vi "Save.vi"(8 "error in":errorcluster) -> (0 "error out":errorcluster)   [LabVIEW 2015, in "Main INI.lvlib"]
uses:
  Main INI.lvlib
  Action.ctl
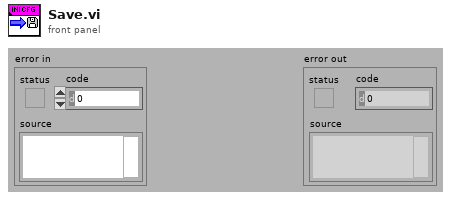
[diagram p1: front panel]
types:
  T1 = typedef "Main INI.lvlib/Action.ctl" = enum16{"Initialise", "Save", "Load", "get All", "set System Config"}
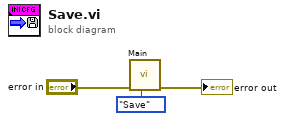
[diagram p0: block diagram]
diagram:
  n1 = call "Main.vi"("Action (get)"=Action."Save", "error in"="error in") -> ("error out"=→"error out":errorcluster)  [unwired: 8 in, 1 out]
